vi "RT Loop - Publish IO.vi"(11 "Message Queue":refnum<queue>) -> ()   [LabVIEW 2017]
uses:
  support/Message Queue/Message Cluster.ctl
  <vilib>/Skyline/Tag/Shared/typedefs/DataType.ctl
  <vilib>/Skyline/Configuration/Configuration AMQP_class/Open Configuration AMQP.vi
  <vilib>/Skyline/Tag/Wrapper/Wrapper AMQP_class/Open Tag AMQP.vi
  <vilib>/Skyline/Tag/Wrapper/Wrapper_class/Generate Tag Cluster (DBL) 2.vi
  <vilib>/Skyline/Configuration/Configuration_class/NI Skyline Configuration.lvclass
  <vilib>/Skyline/Configuration/Configuration HTTP_class/NI Skyline Configuration HTTP.lvclass
  <vilib>/Skyline/Configuration/Configuration AMQP_class/NI Skyline Configuration AMQP.lvclass
  <vilib>/Skyline/Tag/Wrapper/Wrapper_class/NI Skyline Tag.lvclass
  <vilib>/Skyline/Tag/Shared/NI Skyline Tag.lvlib
  <vilib>/Skyline/Tag/Wrapper/Wrapper AMQP_class/NI Skyline Tag AMQP.lvclass
  support/Message Queue/Message Queue.lvlib
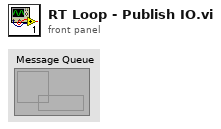
[diagram p1: front panel]
types:
  T1 = typedef "NI Skyline Tag.lvlib/DataType.ctl" = enum32{"Double", "Integer", "String"}
  T2 = typedef "NI Skyline Tag.lvclass/Tag Value Cluster Wrapper.ctl" = cluster{"Configuration":refnum<class "NI Skyline Configuration.lvclass">, "Tag Cluster":T3}
  T3 = typedef "NI Skyline Tag.lvlib/Tag Value Cluster.ctl" = cluster{"Path":string, "Data Type":T1, "Value":string, "Time Stamp":timestamp}
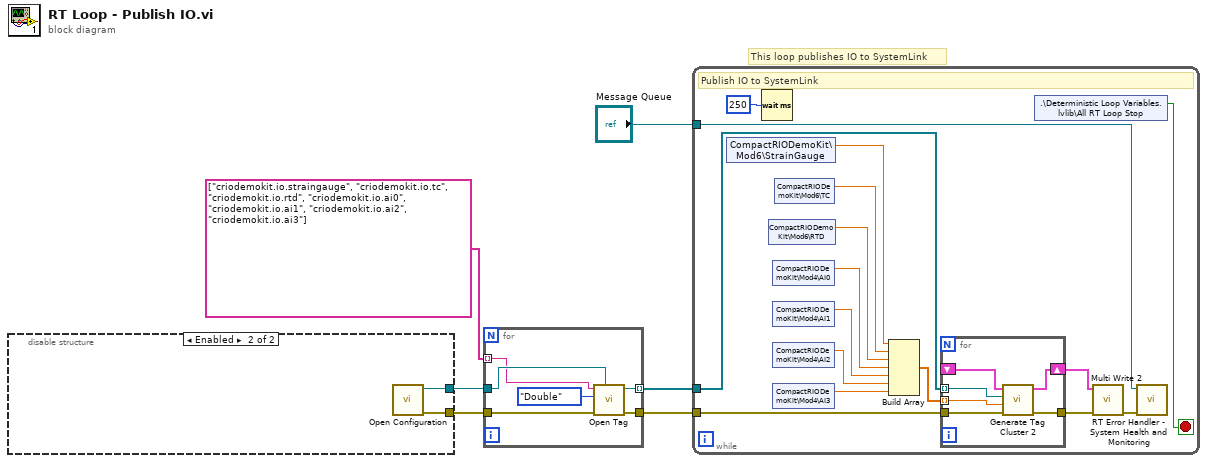
[diagram p0: block diagram]
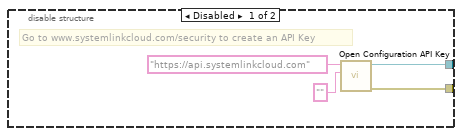
[diagram p2: hidden frame]
diagram:
  # "This loop publishes IO to SystemLink"
  n1 = disable-structure shown="Enabled" {
    disable-tunnel: [w8 w12] -> w5
    disable-tunnel: [w7 w11] -> w3
    frame Disabled {
      # "Go to www.systemlinkcloud.com/security to create an API Key"
      n2 = call <vilib>:"Open Configuration API Key.vi"("api key"="", "server url"="https://api.systemlinkcloud.com") -> ("error out"=w7:errorcluster, "HTTP configuration out"=w8:refnum<class "NI Skyline Configuration HTTP.lvclass">)  [unwired: 8 in]
    }
    frame Enabled {
      n3 = call-poly <vilib>:"Open Configuration.vi"() -> ("error out"=w11:errorcluster, "AMQP configuration out"=w12:refnum<class "NI Skyline Configuration AMQP.lvclass">)  [unwired: 10 in]
    }
  }
  n4 = for {
    tunnel: w5 -> [w18]
    tunnel: string[] ["criodemokit.io.straingauge", "criodemokit.io.tc", "criodemokit.io.rtd", "criodemokit.io.ai0", "criodemokit.io.ai1", "criodemokit.io.ai2", "criodemokit.io.ai3"] -> [w16] mode=indexing
    tunnel: w3 -> [w15]
    tunnel: [w14] -> w2
    tunnel: [w13] -> w1 mode=indexing
    n5 = call-poly <vilib>:"Open Tag.vi"("configuration"=w18, "error in (no error)"=w15, "data type"=DataType."Double", "path"=w16) -> ("error out"=w14:errorcluster, "tag out"=w13:refnum<class "NI Skyline Tag.lvclass">)  [unwired: 6 in]
  }
  n6 = while {
    tunnel: "Message Queue" -> [w19]
    tunnel: w2 -> [w23]
    tunnel: w1 -> [w26]
    stop <- w34 stop-if-true
    # "Publish IO to SystemLink"
    n7 = shared-variable "CompactRIODemoKit\\Mod6\\StrainGauge"() -> (w33:dbl)  [unwired: 1 in, 1 out]
    n8 = Wait (ms)(milliseconds to wait=u32 250) -> ()  [unwired: 1 out]
    n9 = shared-variable "CompactRIODemoKit\\Mod6\\RTD"() -> (w31:dbl)  [unwired: 1 in, 1 out]
    n10 = shared-variable "CompactRIODemoKit\\Mod4\\AI0"() -> (w30:dbl)  [unwired: 1 in, 1 out]
    n11 = shared-variable "CompactRIODemoKit\\Mod4\\AI1"() -> (w29:dbl)  [unwired: 1 in, 1 out]
    n12 = shared-variable "CompactRIODemoKit\\Mod4\\AI2"() -> (w28:dbl)  [unwired: 1 in, 1 out]
    n13 = shared-variable "CompactRIODemoKit\\Mod4\\AI3"() -> (w27:dbl)  [unwired: 1 in, 1 out]
    n14 = shared-variable "CompactRIODemoKit\\Mod6\\TC"() -> (w32:dbl)  [unwired: 1 in, 1 out]
    n15 = Build Array(w33, w32, w31, w30, w29, w28, w27) -> (w22:dbl[])
    n16 = for {
      tunnel: w26 -> [w40] mode=indexing
      shift-right: [w39] -> w25
      shift-left: _ -> [w38]
      tunnel: [w37] -> w24
      tunnel: w23 -> [w36]
      tunnel: w22 -> [w35] mode=indexing
      n17 = call-poly <vilib>:"Generate Tag Cluster 2.vi"("error in (no error)"=w36, "value"=w35, "tag in"=w40, "tag clusters in"=w38) -> ("error out"=w37:errorcluster, "tag clusters out"=w39:T2[])  [unwired: 5 in, 1 out]
    }
    n18 = shared-variable ".\\Deterministic Loop Variables.lvlib\\All RT Loop Stop"() -> (w34:bool)  [unwired: 1 in, 1 out]
    n19 = call <vilib>:"Multi Write 2.vi"("error in (no error)"=w24, "tag clusters"=w25) -> ("error out"=w20:errorcluster)  [unwired: 9 in]
    n20 = call "RT Error Handler - System Health and Monitoring.vi"("error in (no error)"=w20, "Message Queue"=w19) -> ()  [unwired: 9 in, 1 out]
  }
